vi "add_TransformStamped.vi"(4 "Transform":T1, 5 "child_frame_id":string, 6 "Stamp":cluster{"frame_id":string, "reset seq?":bool}, 7 "msg in":string) -> (3 "msg out":string)   [LabVIEW 2014]
doc: "Flattens a transform stamped into a message"
uses:
  std_msgs/subs/stringScalar.vi
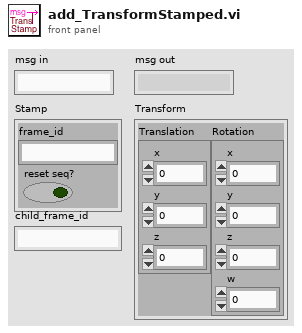
[diagram p1: front panel]
types:
  T1 = cluster{"Translation":cluster{"x":dbl, "y":dbl, "z":dbl}, "Rotation":cluster{"x":dbl, "y":dbl, "z":dbl, "w":dbl}}
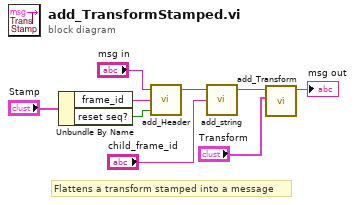
[diagram p0: block diagram]
diagram:
  # "Flattens a transform stamped into a message"
  n1 = Unbundle By Name("Stamp") -> ("frame_id"=w2:string, "reset seq?"=w1:bool)
  n2 = call "add_Header.vi"("reset seq?"=w1, "frame_id"=w2, "msg in"="msg in") -> ("msg out"=w7:string)  [unwired: 2 in]
  n3 = call-poly "add_string.vi"("String"="child_frame_id", "msg in"=w7) -> ("msg out"=w6:string)  [unwired: 3 in]
  n4 = call "add_Transform.vi"("Transform"="Transform", "msg in"=w6) -> ("msg out"=→"msg out":string)  [unwired: 5 in]
